vi "TLA_boxing Suba.vi"(0 "Traceability 引用句柄":refnum<k24>, 1 "StationID":i32, 2 "toBoxQty":i32, 5 "boxBarcode":string, 7 "JobNo":string, 9 "ProcessID":i32, 11 "error in (no error)":errorcluster caption="错误输入（无错误）", 12 "SubaName":string, 13 "User":string) -> (4 "Traceability 引用句柄输出":refnum<k24>, 6 ".NET:System.Data.DataTable":T1 {"RemotingFormat" items=["Xml", "Binary"]}, 15 "error out":errorcluster caption="错误输出")   [LabVIEW 2014, in "Traceability.lvlib"]
uses:
  D:/webservice/Traceability.dll
  Traceability.dll
  System.Data
  Traceability.lvlib
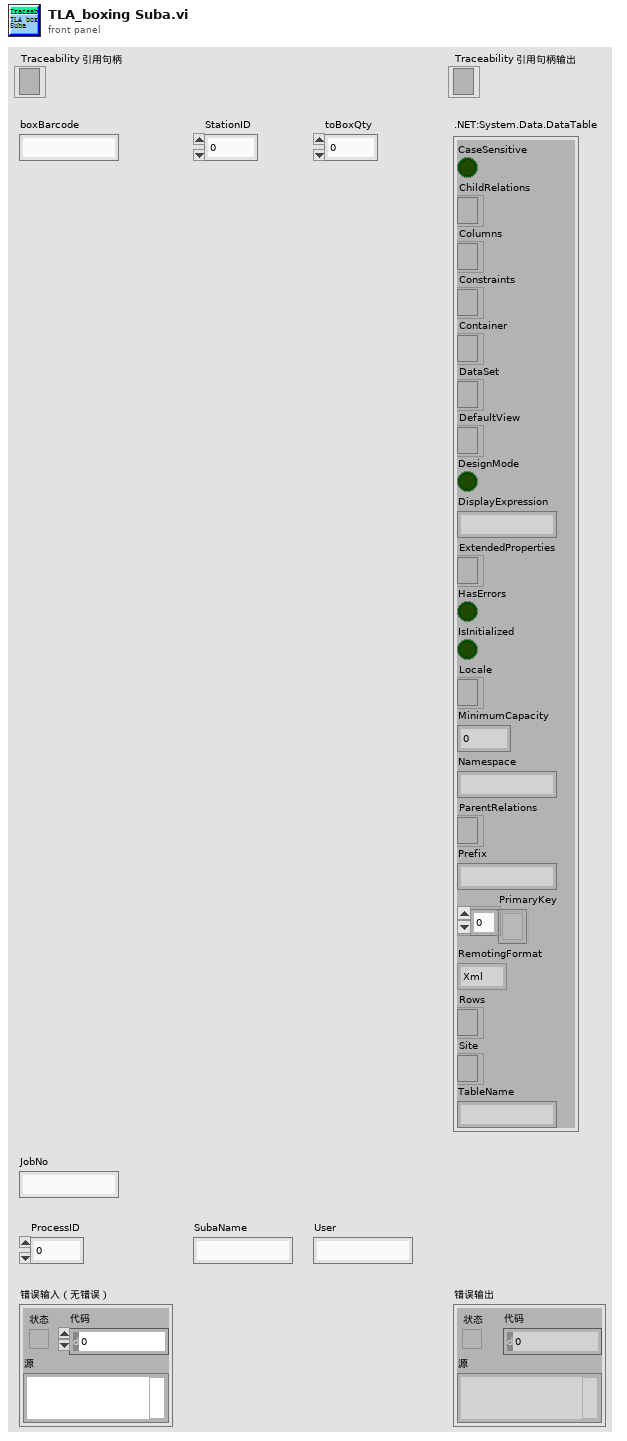
[diagram p1: front panel]
types:
  T1 = cluster{"CaseSensitive":bool, "ChildRelations":refnum<k24>, "Columns":refnum<k24>, "Constraints":refnum<k24>, "Container":refnum<k24>, "DataSet":refnum<k24>, "DefaultView":refnum<k24>, "DesignMode":bool, "DisplayExpression":string, "ExtendedProperties":refnum<k24>, "HasErrors":bool, "IsInitialized":bool, "Locale":refnum<k24>, "MinimumCapacity":i32, "Namespace":string, "ParentRelations":refnum<k24>, "Prefix":string, "PrimaryKey":refnum<k24>[], "RemotingFormat":i32, "Rows":refnum<k24>, "Site":refnum<k24>, "TableName":string}
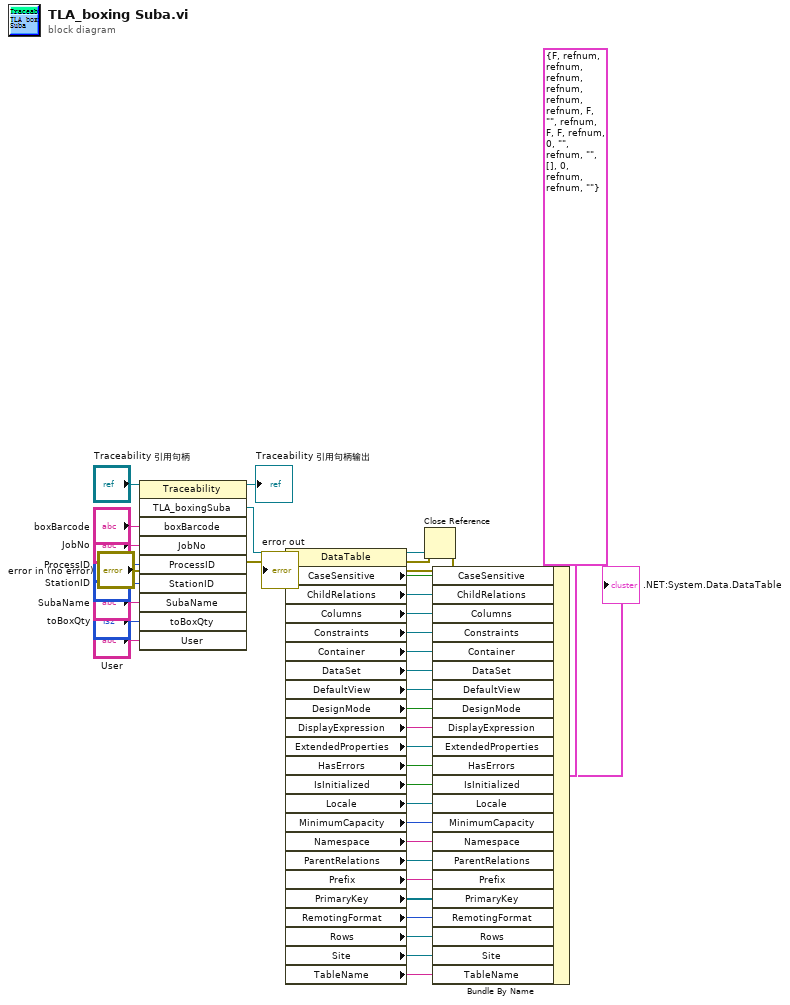
[diagram p0: block diagram]
diagram:
  n1 = invoke class="Traceability" method="TLA_boxingSuba"(reference="Traceability 引用句柄", error in="error in (no error)", "boxBarcode"="boxBarcode", "JobNo"="JobNo", "ProcessID"="ProcessID", "StationID"="StationID", "SubaName"="SubaName", "toBoxQty"="toBoxQty", "User"="User") -> (reference out=→"Traceability 引用句柄输出":refnum<k24>, error out=w4:errorcluster, "TLA_boxingSuba"=w36:refnum<k24>)  [unwired: 1 in, 7 out]
  n2 = property class="DataTable"(reference=w36, error in=w4) -> (reference out=w3:refnum<k24>, error out=w2:errorcluster, "CaseSensitive"=w33:bool, "ChildRelations"=w32:refnum<k24>, "Columns"=w31:refnum<k24>, "Constraints"=w30:refnum<k24>, "Container"=w29:refnum<k24>, "DataSet"=w28:refnum<k24>, "DefaultView"=w27:refnum<k24>, "DesignMode"=w26:bool, "DisplayExpression"=w25:string, "ExtendedProperties"=w24:refnum<k24>, "HasErrors"=w23:bool, "IsInitialized"=w22:bool, "Locale"=w21:refnum<k24>, "MinimumCapacity"=w20:i32, "Namespace"=w19:string, "ParentRelations"=w18:refnum<k24>, "Prefix"=w17:string, "PrimaryKey"=w16:refnum<k24>[], "RemotingFormat"=w15:i32, "Rows"=w14:refnum<k24>, "Site"=w13:refnum<k24>, "TableName"=w12:string)
  n3 = Close Reference(reference=w3, error in (no error)=w2) -> (error out=→"error out":errorcluster)
  n4 = Bundle By Name(cluster=T1 {"CaseSensitive"=FALSE, "ChildRelations"=refnum, "Columns"=refnum, "Constraints"=refnum, "Container"=refnum, "DataSet"=refnum, "DefaultView"=refnum, "DesignMode"=FALSE, "DisplayExpression"="", "ExtendedProperties"=refnum, "HasErrors"=FALSE, "IsInitialized"=FALSE, "Locale"=refnum, "MinimumCapacity"=0, "Namespace"="", "ParentRelations"=refnum, "Prefix"="", "PrimaryKey"=[], "RemotingFormat"=0, "Rows"=refnum, "Site"=refnum, "TableName"=""} (".NET:System.Data.DataTable"), "CaseSensitive"=w33, "ChildRelations"=w32, "Columns"=w31, "Constraints"=w30, "Container"=w29, "DataSet"=w28, "DefaultView"=w27, "DesignMode"=w26, "DisplayExpression"=w25, "ExtendedProperties"=w24, "HasErrors"=w23, "IsInitialized"=w22, "Locale"=w21, "MinimumCapacity"=w20, "Namespace"=w19, "ParentRelations"=w18, "Prefix"=w17, "PrimaryKey"=w16, "RemotingFormat"=w15, "Rows"=w14, "Site"=w13, "TableName"=w12) -> (→".NET:System.Data.DataTable":T1)
